vi "_Reentrant Measurement.vi"() -> ()   [LabVIEW 2021, in "MeasurementServerTests.lvlib" / "Measurement Service Tests.lvlib" / "Continuous Counting Measurement.lvclass"]
uses:
  Continuous Counting Measurement.lvclass
  Runtime/Measurements/Measure Call Context/Measure Call Context.lvclass
  Measurement Configuration.ctl
  Measurement Results.ctl
panel:
  out "measurement results":T1
  in  "measurement configuration":T2
  out "error out":errorcluster
  in  "error in":errorcluster
  out "measure call context out":refnum<class "Measure Call Context.lvclass">
  in  "measure call context in":refnum<class "Measure Call Context.lvclass">
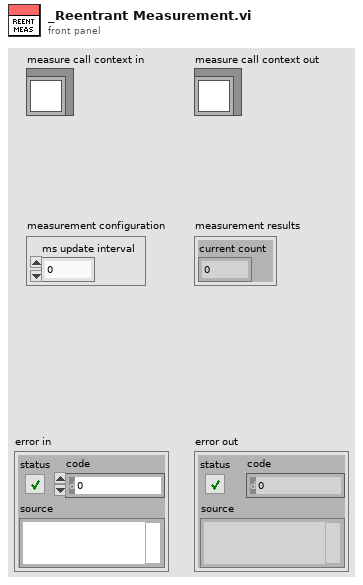
[diagram p1: front panel]
types:
  T1 = typedef "MeasurementServerTests.lvlib/Measurement Service Tests.lvlib/Continuous Counting Measurement.lvclass/Measurement Results.ctl" = cluster{"current count":i64}
  T2 = typedef "MeasurementServerTests.lvlib/Measurement Service Tests.lvlib/Continuous Counting Measurement.lvclass/Measurement Configuration.ctl" = cluster{"ms update interval":u32}
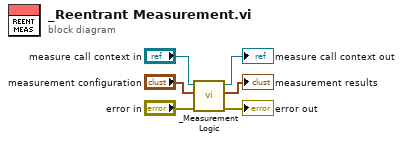
[diagram p0: block diagram]
diagram:
  n1 = call "_Measurement Logic.vi"("error in"="error in", "measurement configuration"="measurement configuration", "measure call context in"="measure call context in") -> ("error out"=→"error out":errorcluster, "measurement results"=→"measurement results":T1, "measure call context out"=→"measure call context out":refnum<class "Measure Call Context.lvclass">)  [unwired: 6 in]
